vi "Open Playback Files.vi"(8 "error in (no error)":errorcluster, 11 "Frame Grabber Data In":T1) -> (0 "error out":errorcluster, 1 "Playback Video":path, 2 "both exist and open?":bool, 3 "Frame Grabber Data Out":T1, 4 "Gestation":string)   [LabVIEW 2017]
uses:
  Controls/Frame Grabber Data.ctl
  <vilib>/userdefined/High Color/IMAQdx.ctl
  <vilib>/vision/Image Controls.llb/IMAQ Image.ctl
  <vilib>/vision/Avi.llb/IMAQ AVI2 Refnum.ctl
  Controls/Rigid Body Info.ctl
  Controls/Position.ctl
  Controls/Orientation.ctl
  <userlib>/_OpenG.lib/file/file.llb/File Exists - Scalar__ogtk.vi
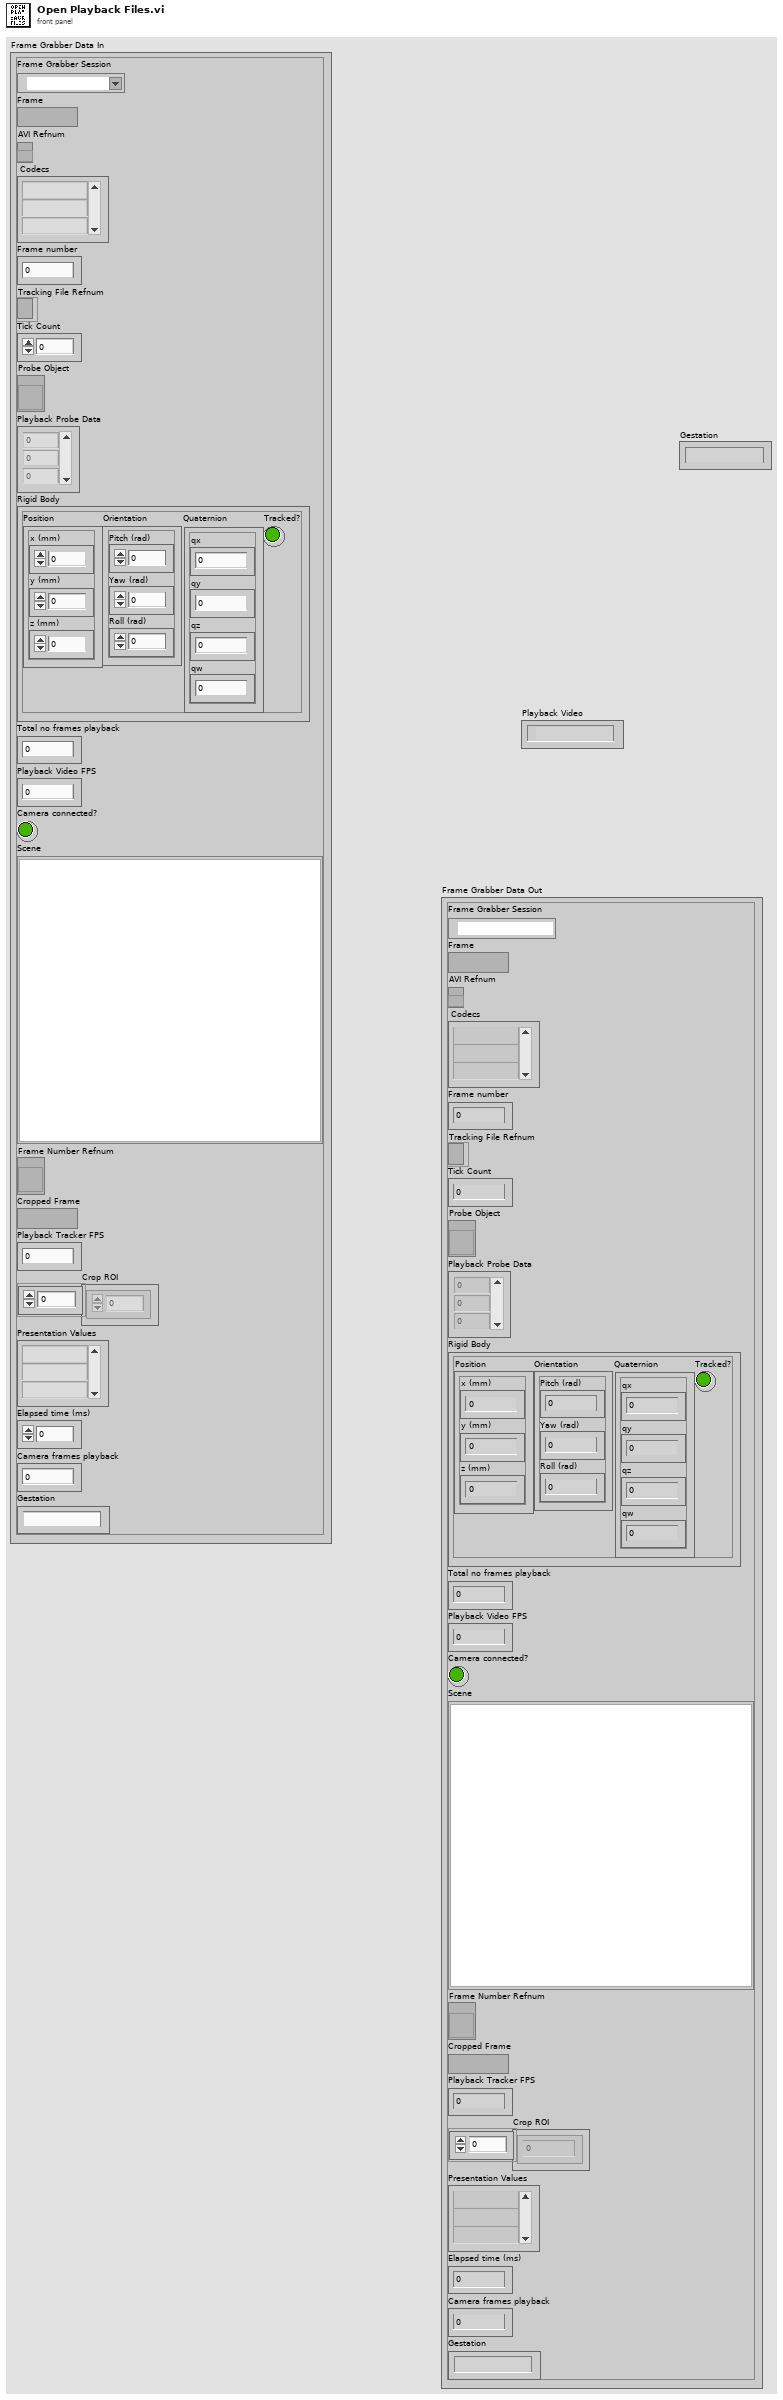
[diagram p1: front panel]
types:
  T1 = typedef "Frame Grabber Data.ctl" = cluster{"Camera Session":T2, "Frame":T3, "AVI Refnum":T4, "Codecs":string[], "Frame number":u32, "Tracking File Refnum":refnum<file>, "Tick Count":u32, "Probe Object":refnum<vi>, "Playback Probe Data":dbl[][], "Rigid Body":T5, "Total no frames playback":u32, "Playback Video FPS":u32, "Camera connected?":bool, "Scene":refnum<vi>, "Frame Number Refnum":refnum<vi>, "Cropped Frame":T3, "Playback Tracker FPS":u32, "Crop ROI":i32[], "Presentation Values":string[], "Elapsed time (ms)":u32, "Camera frames playback":u32, "Gestation":string}
  T2 = typedef "IMAQdx.ctl" = refnum<k21>
  T3 = typedef "IMAQ Image.ctl" = refnum<image>
  T4 = typedef "IMAQ AVI2 Refnum.ctl" = refnum<k20>
  T5 = typedef "Rigid Body Info.ctl" = cluster{"Position":T6, "Orientation":T7, "Quaternion":cluster{"qx":sgl, "qy":sgl, "qz":sgl, "qw":sgl}, "Tracked?":bool}
  T6 = typedef "Position.ctl" = cluster{"x (mm)":sgl, "y (mm)":sgl, "z (mm)":sgl}
  T7 = typedef "Orientation.ctl" = cluster{"Pitch (rad)":sgl, "Yaw (rad)":sgl, "Roll (rad)":sgl}
  T8 = enum16{"open", "replace", "create", "open or create", "replace or create", "replace or create with confirmation"}
  T9 = cluster{"Width":u32, "Height":u32, "Frames Per Second":u32, "Codec":string, "Has Data":bool}
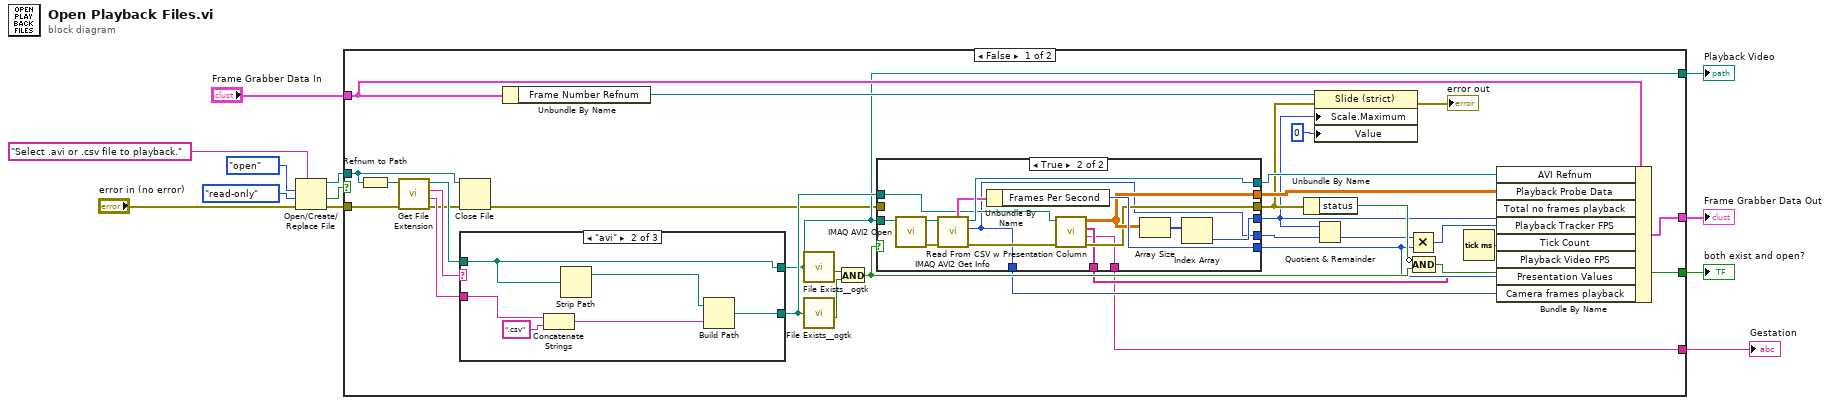
[diagram p0: block diagram]
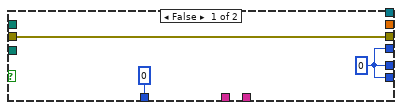
[diagram p2: hidden frame]
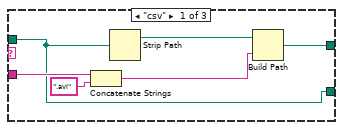
[diagram p3: hidden frame]
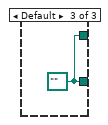
[diagram p4: hidden frame]
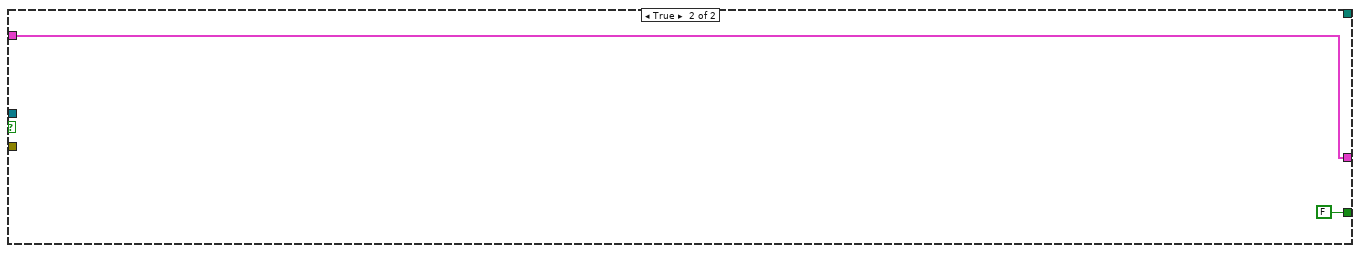
[diagram p5: hidden frame]
diagram:
  n1 = Open/Create/Replace File(error in="error in (no error)", prompt="Select .avi or .csv file to playback.", operation (0:open)=T8."open", access (0:read/write)=enum16{"read/write", "read-only", "write-only"}."read-only") -> (refnum out=w10:refnum<file>, cancelled=w3:bool, error out=w12:errorcluster)  [unwired: 2 in]
  n2 = case shown="False" w3 {
    tunnel: w12 -> [w44 _]
    tunnel: w10 -> [w17 _]
    tunnel: "Frame Grabber Data In" -> [w27 w77]
    tunnel: [w33 FALSE] -> w5
    tunnel: [w31 w77] -> w4
    tunnel: [w24 _] -> w2
    tunnel: [w13 _] -> w1
    frame False {
      n3 = Refnum to Path(1:w17) -> (0:w43:path)
      n4 = call <vilib>:"Get File Extension.vi"("error in (no error)"=w44, "file"=w43) -> ("error out"=w19:errorcluster, "filename without extension"=w41:string, "lowercase file extension"=w42:string, "dup file"=w40:path)  [unwired: 5 in, 1 out]
      n5 = Close File(refnum=w17, error in=w19) -> (error out=w18:errorcluster)  [unwired: 1 out]
      n6 = case shown="\"avi\"" w42 {
        tunnel: w41 -> [w68 w73 _]
        tunnel: w40 -> [w65 w72 _]
        tunnel: [w63 w72 w75] -> w24
        tunnel: [w65 w69 w75] -> w37
        frame "csv" {
          n7 = Concatenate Strings(w68, ".avi" ("string")) -> (w64:string)
          n8 = Strip Path(path=w65) -> (stripped path=w66:path)  [unwired: 1 out]
          n9 = Build Path(base path=w66, name or relative path=w64) -> (appended path=w63:path)
        }
        frame "avi" {
          n10 = Concatenate Strings(w73, ".csv" ("string")) -> (w70:string)
          n11 = Strip Path(path=w72) -> (stripped path=w71:path)  [unwired: 1 out]
          n12 = Build Path(base path=w71, name or relative path=w70) -> (appended path=w69:path)
        }
        frame Default {
          w75 = path "" ("dup file")
        }
      }
      n13 = Unbundle By Name(w27) -> ("Frame Number Refnum"=w26:refnum<vi>)
      n14 = call-poly <userlib>:"File Exists__ogtk.vi"("file path"=w24) -> ("exists"=w35:bool)  [unwired: 6 in, 1 out]
      n15 = call-poly <userlib>:"File Exists__ogtk.vi"("file path"=w37) -> ("exists"=w36:bool)  [unwired: 6 in, 1 out]
      n16 = And(x=w35, y=w36) -> (x .and. y?=w34:bool)
      n17 = case shown="True" w34 {
        tunnel: w18 -> [w47 _]
        tunnel: w24 -> [_ w62]
        tunnel: [w47 w54] -> w29
        tunnel: [_ w59] -> w39
        tunnel: [_ w56] -> w38
        tunnel: w37 -> [_ w51]
        tunnel: [w46 w49] -> w20
        tunnel: [w46 w57] -> w21
        tunnel: [w46 w52] -> w16
        tunnel: [_ w50] -> w15
        tunnel: [u32 0 ("Number of Frames") w49] -> w14
        tunnel: [_ w48] -> w13
        frame False {
          w46 = u32 0 ("Number of Frames")
        }
        frame True {
          n18 = call "IMAQ AVI2 Open"("AVI File Path"=w62) -> ("error out"=w61:errorcluster, "AVI Refnum"=w60:T4)  [unwired: 9 in]
          n19 = call "IMAQ AVI2 Get Info"("error in (no error)"=w61, "AVI Refnum"=w60) -> ("error out"=w55:errorcluster, "Number of Frames"=w49:u32, "AVI Refnum (duplicate)"=w59:T4, "Frame Data"=w58:T9)  [unwired: 5 in, 1 out]
          n20 = Unbundle By Name(w58) -> ("Frames Per Second"=w57:u32)
          n21 = call "Read From CSV w Presentation Column.vi"("Error In"=w55, "Spreadsheet path (.csv)"=w51) -> ("Error Out"=w54:errorcluster, "Gestation"=w48:string, "Presentation Values"=w50:string[], "Data"=w56:dbl[][])  [unwired: 6 in]
          n22 = Array Size(array=w56) -> (size(s)=w53:i32[])
          n23 = Index Array(array=w53) -> (element=w52:i32)  [unwired: 1 in]
        }
      }
      n24 = Unbundle By Name(w29) -> ("status"=w32:bool)
      n25 = property class="Slide (strict)"(reference=w26, error in=w29, "Scale.Maximum"=w16, "Value"=u32 0 ("Frame number")) -> (error out=→"error out":errorcluster)  [unwired: 1 out]
      n26 = Quotient & Remainder(x=w16, y=w20) -> (floor(x/y)=w23:u32)  [unwired: 1 out]
      n27 = Multiply(x=w23, y=w21) -> (x*y=w22:u32)
      n28 = Compound Arithmetic op=AND(invert w32, w34) -> (w33:bool)
      n29 = Tick Count (ms)() -> (millisecond timer value=w30:u32)
      n30 = Bundle By Name(cluster=w27, "AVI Refnum"=w39, "Playback Probe Data"=w38, "Total no frames playback"=w16, "Playback Tracker FPS"=w22, "Tick Count"=w30, "Playback Video FPS"=w21, "Presentation Values"=w15, "Camera frames playback"=w14) -> (w31:T1)
    }
    frame True {
    }
  }
  "both exist and open?" <- w5
  "Frame Grabber Data Out" <- w4
  "Playback Video" <- w2
  "Gestation" <- w1
